vi "OAT Waterfall Compute Plots.vi"(4 "zoom factor":i32=5, 6 "Y axis offset":i32, 7 "Y scale":cluster{"offset":dbl, "multiplier":dbl} {"multiplier" format="%.2f"; "offset" format="%.2f"}, 8 "max Z range":dbl=5.0 format="%.2e", 9 "plot settings":T1={"plot color"=0, "grid color"=0, "X shift (rel to total X)"=0.1, "max Z range"=11, "number of spectra"=40} {"max Z range" items=["10^-7", "10^-6", "10^-5", "0.0001", "0.001", "0.01", "0.1", "1", "10", "100", "1000", "auto z range"]; "X shift (rel to total X)" format="%.2f"}, 10 "spectral map in":dbl[][](array[numeric]) format="%.2f", 11 "X scale":cluster{"offset":dbl, "multiplier":dbl} {"multiplier" format="%.2f"; "offset" format="%.2f"}) -> (0 "max x axis offset":dbl, 1 "# of bins":i32, 2 "spectral map out":dbl[][](array[numeric]) format="%.2f", 3 "waterfall plot":cluster{"X0":dbl, "dX":dbl, "Y":dbl[]}[](array[cluster]) {"Y" format="%.2f"; "dX" format="%.2f"; "X0" format="%.2f"})   [LabVIEW 2017]
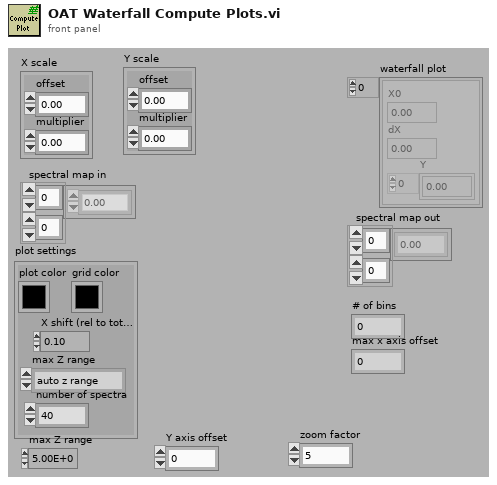
[diagram p1: front panel]
types:
  T1 = cluster{"plot color":u32, "grid color":u32, "X shift (rel to total X)":dbl, "max Z range":u16, "number of spectra":i32}
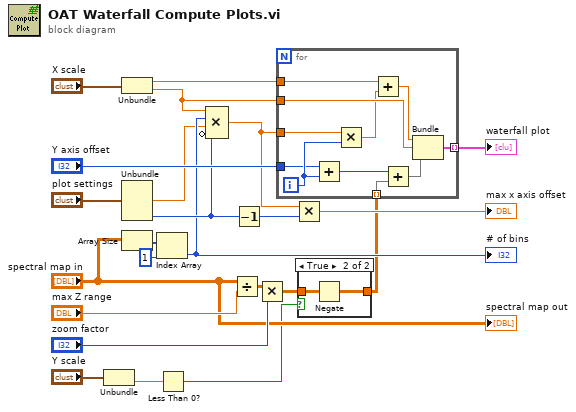
[diagram p0: block diagram]
diagram:
  n1 = Unbundle("Y scale") -> ("multiplier"=w4:dbl)  [unwired: 1 out]
  n2 = Unbundle("X scale") -> ("offset"=w19:dbl, "multiplier"=w16:dbl)
  n3 = Unbundle("plot settings") -> ("X shift (rel to total X)"=w7:dbl, "number of spectra"=w10:i32)  [unwired: 3 out]
  n4 = Array Size(array="spectral map in") -> (size(s)=w14:i32[])
  n5 = Index Array(array=w14, index=1) -> (element=w9:i32)
  "# of bins" <- w9
  n6 = Less Than 0?(x=w4) -> (x < 0?=w3:bool)
  n7 = Compound Arithmetic op=MULTIPLY(w16, w9, w7, invert w10) -> (w12:dbl)
  n8 = Divide(x="spectral map in", y="max Z range") -> (x/y=w22:dbl[][])
  n9 = Decrement(x=w10) -> (x-1=w6:i32)
  n10 = Multiply(x=w22, y="zoom factor") -> (x*y=w2:dbl[][])
  n11 = Multiply(x=w12, y=w6) -> (x*y=→"max x axis offset":dbl)
  n12 = case shown="True" w3 {
    tunnel: w2 -> [w24 w26]
    tunnel: [w24 w25] -> w1
    frame False {
    }
    frame True {
      n13 = Negate(x=w26) -> (-x=w25:dbl[][])
    }
  }
  n14 = for {
    tunnel: w12 -> [w37]
    tunnel: w19 -> [w36]
    tunnel: w16 -> [w34]
    tunnel: [w33] -> w18 mode=indexing
    tunnel: "Y axis offset" -> [w31]
    tunnel: w1 -> [w27] mode=indexing
    i -> [w32]
    n15 = Add(x=w31, y=w32) -> (x+y=w29:i32)
    n16 = Multiply(x=w37, y=w32) -> (x*y=w30:dbl)
    n17 = Add(x=w36, y=w30) -> (x+y=w35:dbl)
    n18 = Add(x=w29, y=w27) -> (x+y=w28:dbl[])
    n19 = Bundle(w35, "multiplier"=w34, w28) -> (w33:cluster{dbl, "multiplier":dbl, dbl[]})  [unwired: 1 in]
  }
  "waterfall plot" <- w18
  "spectral map out" <- "spectral map in"
